vi "ScanFeedback.vi"(2 "measurement type":T1(tab)) -> (1 "V breakdown":dbl, 5 "V depletion":dbl, 6 "Maximum current fluctuations [%]":dbl[](array[numeric]), 8 "Ris [MOhm]":dbl, 9 "Cis @300V [pF/cm]":dbl)   [LabVIEW 2018]
uses:
  globals/QC_MeasurementSetup.vi
  globals/QC_RunInformation.vi
  <vilib>/Analysis/NI_AALPro.lvlib
  <vilib>/Analysis/NI_AALBase.lvlib
panel:
  out "MEAN":dbl
  out "STD":dbl
  out "Index lin fit 1":dbl
  out "Slope":dbl
  out "capSquare1":dbl[](array[numeric])
  out "volts1":dbl[](array[numeric])
  out "volts2":dbl[](array[numeric])
  out "capSquare2":dbl[](array[numeric])
  out "deriv":dbl[](array[numeric])
  out "Slope 2":dbl
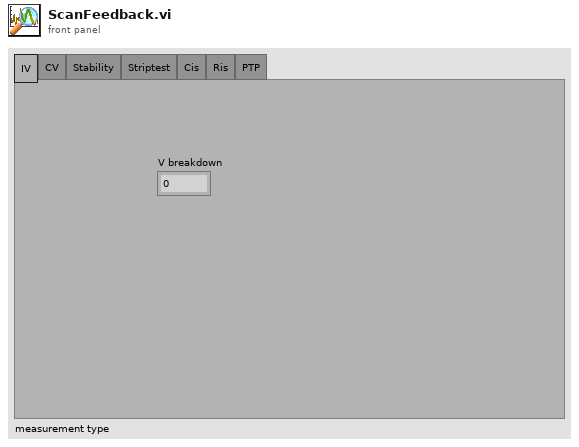
[diagram p1: front panel]
types:
  T1 = enum32{"IV", "CV", "Stability", "Striptest", "Cis", "Ris", "PTP"}
  T2 = enum16{"Reset", "Read Array", "Read Element", "Write Element", "Write Array", "Add Element", "Add Array"}
  T3 = cluster{"Supply":refnum<class "SupplyControl.lvclass">, "Arduino":refnum<class "ArduinoControl.lvclass">, "Measurement switch":refnum<class "Switching.lvclass">, "Initial Voltage [V]":dbl, "Final Voltage [V]":dbl, "Step Size [V]":dbl, "Step Interval [s]":i32, "Number Of Steps":u32, "Ramp down steps [V]":dbl, "Ramp down Interval [s]":i32, "hold steps":i32, "Set Current Limit?":bool, "Current Limit [µA]":dbl, "Temperature Readout":enum16{"Read Arduino", "Enter manually"}, "Supply Name":string, "V_breakdown Limit [V]":dbl, "Measurement switch used?":bool}
  T4 = cluster{"Sensor Serial No.:":string, "Wafer:":string, "Batch:":string, "Manufacturer:":string, "Device Category:":string, "Database Serial No.:":string, "Date Initiated:":string, "Time Initiated:":string, "Test":string, "Probeplan used:":string, "End of Run comment:":string, "User:":string, "Vbias SMU":string, "LCR":string, "Test SMU":string, "Test DMM":string, "Comments":string}
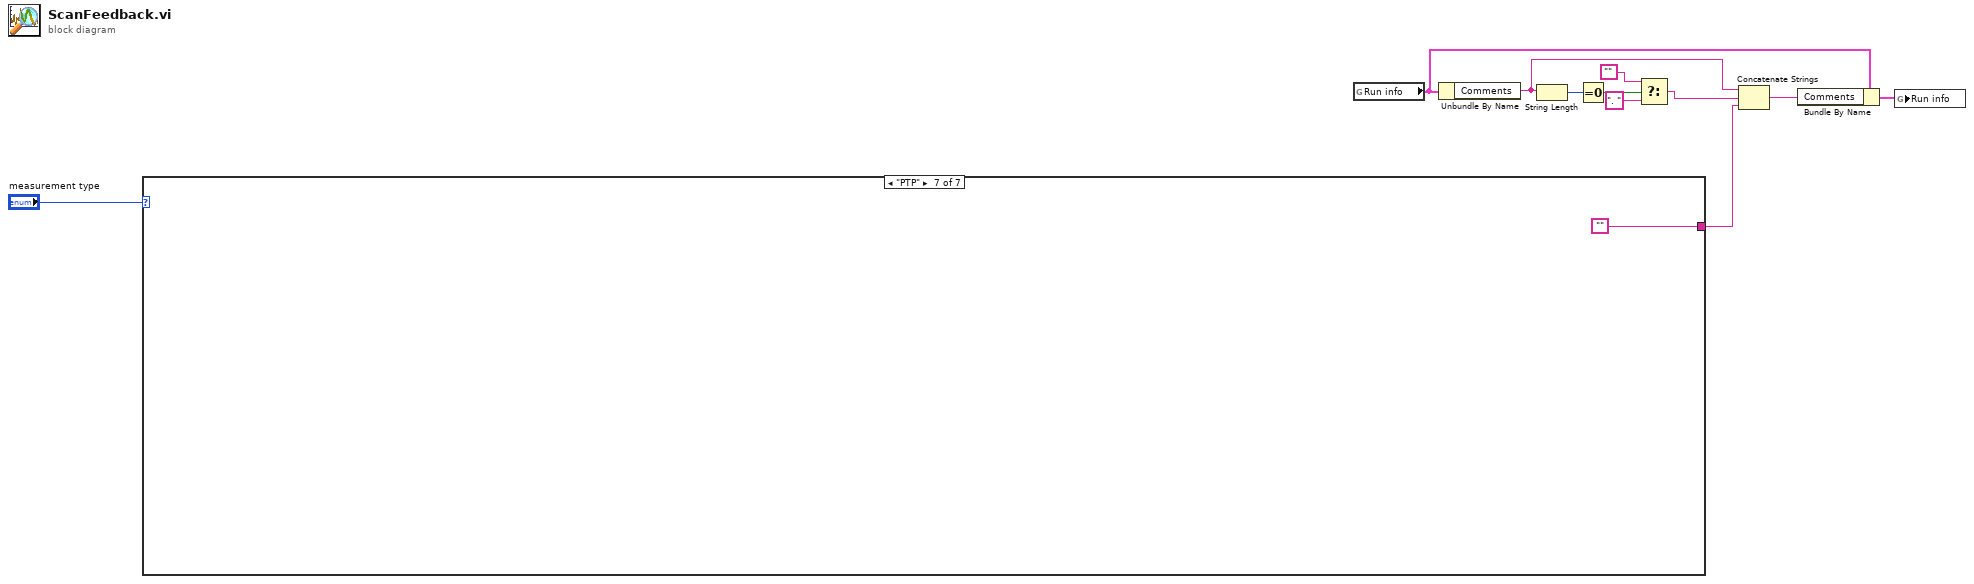
[diagram p0: block diagram]
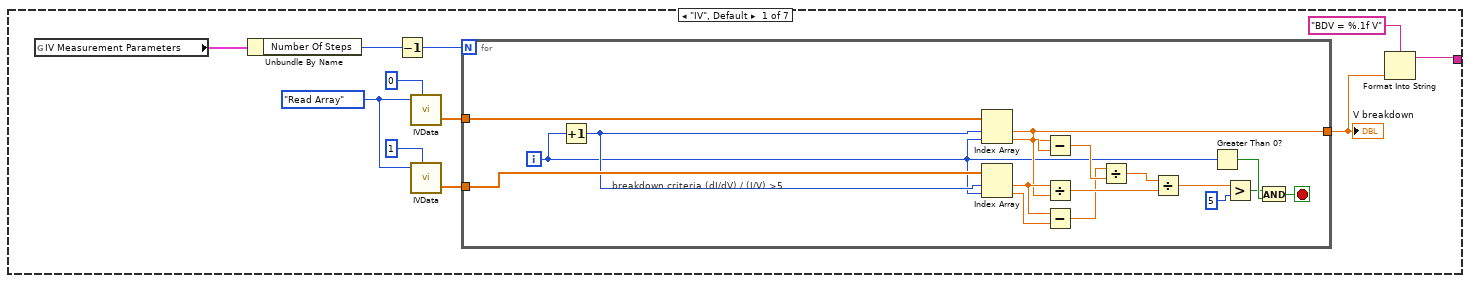
[diagram p2: hidden frame]
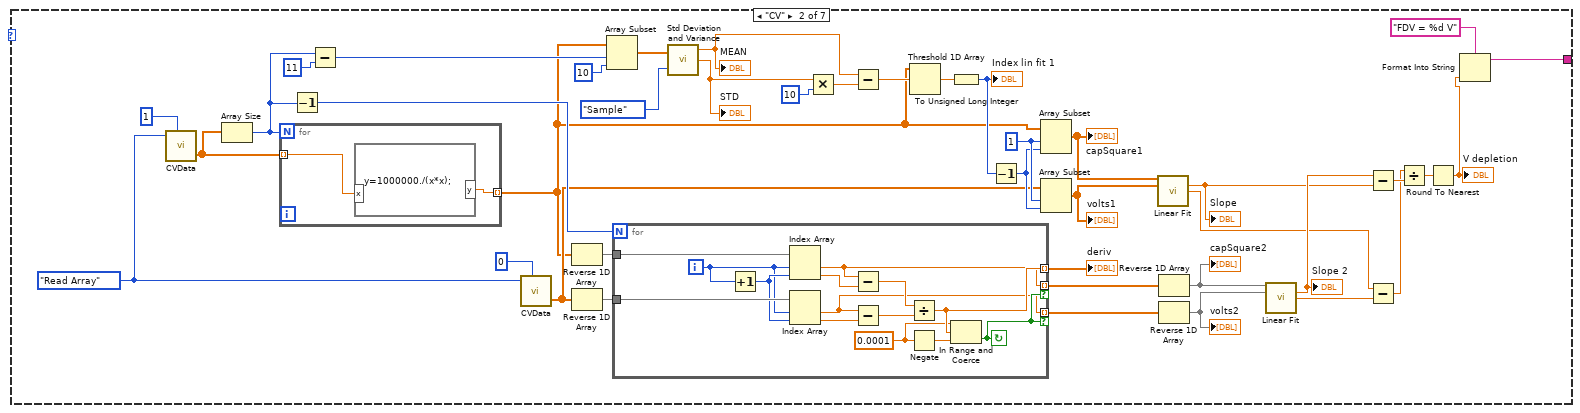
[diagram p3: hidden frame]
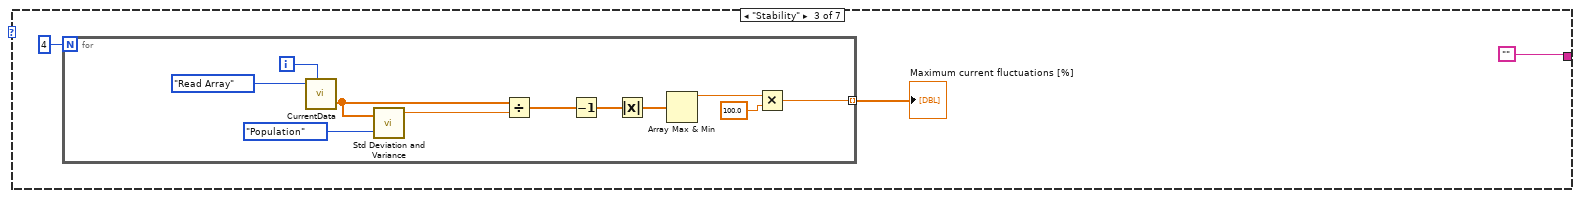
[diagram p4: hidden frame]
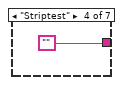
[diagram p5: hidden frame]
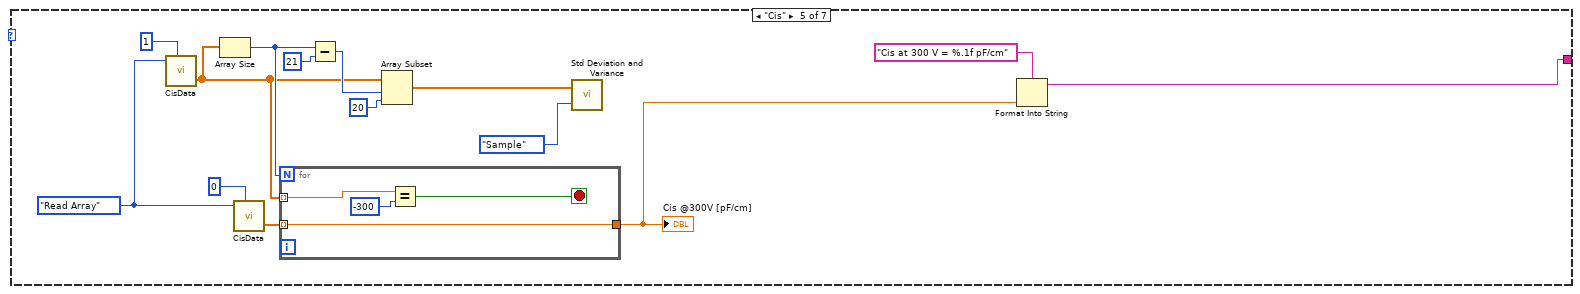
[diagram p6: hidden frame]
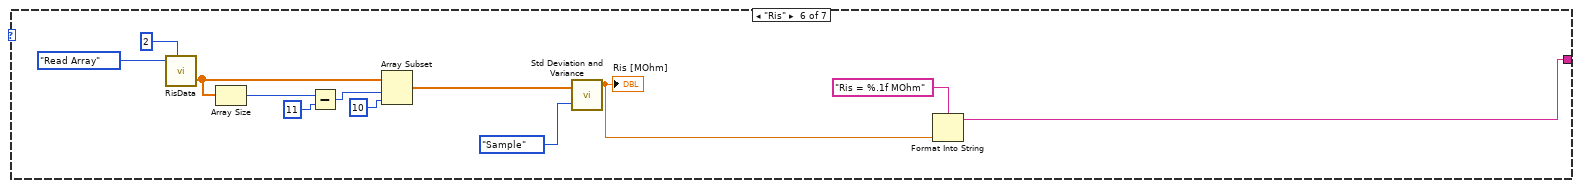
[diagram p7: hidden frame]
diagram:
  n1 = case shown="\"PTP\"" "measurement type" {
    tunnel: [w12 w40 "" "" w112 w130 ""] -> w4
    frame "IV", Default {
      w20 = T2."Read Array" ("Action")
      n2 = global read "QC_MeasurementSetup.vi" "IV Measurement Parameters"() -> (w16:T3)
      n3 = Unbundle By Name(w16) -> ("Number Of Steps"=w15:u32)
      n4 = Decrement(x=w15) -> (x-1=w17:u32)
      n5 = call "IVData.vi"("Action"=w20, "Array No."=0) -> ("Array OUT"=w18:dbl[])  [unwired: 3 in, 1 out]
      n6 = call "IVData.vi"("Action"=w20, "Array No."=1) -> ("Array OUT"=w19:dbl[])  [unwired: 3 in, 1 out]
      n7 = for {
        N: w17 -> [_]
        tunnel: w18 -> [w38]
        tunnel: w19 -> [w39]
        tunnel: [w27] -> w13
        i -> [w25]
        stop <- w23 stop-if-true
        # "breakdown criteria (dI/dV) / (I/V) >5"
        n8 = Increment(x=w25) -> (x+1=w35:i32)
        n9 = Index Array(array=w38, index #1=w35, index #2=w25) -> (element #1=w27:dbl, element #2=w37:dbl)
        n10 = Index Array(array=w39, index #1=w35, index #2=w25) -> (element #1=w30:dbl, element #2=w36:dbl)
        n11 = Subtract(x=w27, y=w37) -> (x-y=w32:dbl)
        n12 = Divide(x=w30, y=w27) -> (x/y=w33:dbl)
        n13 = Subtract(x=w30, y=w36) -> (x-y=w31:dbl)
        n14 = Divide(x=w31, y=w32) -> (x/y=w34:dbl)
        n15 = Divide(x=w34, y=w33) -> (x/y=w28:dbl)
        n16 = Greater Than 0?(x=w25) -> (x > 0?=w26:bool)
        n17 = Greater?(x=w28, y=5) -> (0:w24:bool)
        n18 = And(x=w24, y=w26) -> (x .and. y?=w23:bool)
      }
      "V breakdown" <- w13
      n19 = Format Into String(format string="BDV = %.1f V", w13) -> (resulting string=w12:string)  [unwired: 2 in, 1 out]
    }
    frame "CV" {
      w53 = T2."Read Array" ("Action")
      w50 = 1
      n20 = call "CVData.vi"("Action"=w53, "Array No."=1) -> ("Array OUT"=w44:dbl[])  [unwired: 3 in, 1 out]
      n21 = Array Size(array=w44) -> (size(s)=w45:i32)
      n22 = for {
        N: w45 -> [_]
        tunnel: w44 -> [w82] mode=indexing
        tunnel: [w81] -> w43 mode=indexing
        n23 = formula code="y=1000000./(x*x);"("x"=w82) -> ("y"=w81:dbl)
      }
      n24 = Decrement(x=w45) -> (x-1=w65:i32)
      n25 = Subtract(x=w45, y=11) -> (x-y=w79:i32)
      n26 = call "CVData.vi"("Action"=w53, "Array No."=0) -> ("Array OUT"=w47:dbl[])  [unwired: 3 in, 1 out]
      n27 = Reverse 1D Array(array=w43) -> (reversed array=w68:dbl[])
      n28 = Reverse 1D Array(array=w47) -> (reversed array=w46:dbl[])
      n29 = Array Subset(array=w43, index=w79, length=10) -> (w77:dbl[])
      n30 = for {
        N: w65 -> [_]
        tunnel: w68 -> [w96]
        tunnel: [w89] -> w67 mode=indexing if=w90
        tunnel: [w85] -> w64 mode=indexing if=w90
        tunnel: [w93] -> w61 mode=indexing
        tunnel: w46 -> [w88]
        i -> [w86]
        stop <- w90 continue-if-true
        w91 = 0.0001
        n31 = Increment(x=w86) -> (x+1=w87:i32)
        n32 = Index Array(array=w96, index #1=w86, index #2=w87) -> (element #1=w89:dbl, element #2=w94:dbl)
        n33 = Index Array(array=w88, index #1=w86, index #2=w87) -> (element #1=w85:dbl, element #2=w84:dbl)
        n34 = Subtract(x=w89, y=w94) -> (x-y=w95:dbl)
        n35 = Subtract(x=w85, y=w84) -> (x-y=w83:dbl)
        n36 = Divide(x=w95, y=w83) -> (x/y=w93:dbl)
        n37 = Negate(x=w91) -> (-x=w92:dbl)
        n38 = In Range and Coerce(upper limit=w91, x=w93, lower limit=w92) -> (In Range?=w90:bool)  [unwired: 1 out]
      }
      "deriv" <- w61
      n39 = call <vilib>:"Std Deviation and Variance.vi"("X"=w77, "Weighting (Sample)"=enum16{"Sample", "Population"}."Sample") -> ("mean"=w73:dbl, "standard deviation"=w62:dbl)  [unwired: 1 out]
      "MEAN" <- w73
      "STD" <- w62
      n40 = Multiply(x=w62, y=10) -> (x*y=w74:dbl)
      n41 = Subtract(x=w73, y=w74) -> (x-y=w72:dbl)
      n42 = Threshold 1D Array(2:w72, 3:w43) -> (0:w71:dbl)  [unwired: 1 in]
      n43 = To Unsigned Long Integer(number=w71) -> (unsigned 32bit integer=w70:u32)
      "Index lin fit 1" <- w70
      n44 = Decrement(x=w70) -> (x-1=w49:u32)
      n45 = Array Subset(array=w43, index=w50, length=w49) -> (w69:dbl[])
      "capSquare1" <- w69
      n46 = Array Subset(array=w47, index=w50, length=w49) -> (w48:dbl[])
      "volts1" <- w48
      n47 = call <vilib>:"Linear Fit.vi"("Y"=w69, "X"=w48) -> ("slope"=w59:dbl, "intercept"=w57:dbl)  [unwired: 9 in, 3 out]
      "Slope" <- w59
      n48 = Reverse 1D Array(array=w67) -> (reversed array=w66:dbl[])
      "capSquare2" <- w66
      n49 = Reverse 1D Array(array=w64) -> (reversed array=w63:dbl[])
      "volts2" <- w63
      n50 = call <vilib>:"Linear Fit.vi"("Y"=w66, "X"=w63) -> ("slope"=w60:dbl, "intercept"=w58:dbl)  [unwired: 9 in, 3 out]
      "Slope 2" <- w60
      n51 = Subtract(x=w60, y=w59) -> (x-y=w56:dbl)
      n52 = Subtract(x=w57, y=w58) -> (x-y=w55:dbl)
      n53 = Divide(x=w55, y=w56) -> (x/y=w54:dbl)
      n54 = Round To Nearest(number=w54) -> (nearest integer value=w42:dbl)
      "V depletion" <- w42
      n55 = Format Into String(format string="FDV = %d V", w42) -> (resulting string=w40:string)  [unwired: 2 in, 1 out]
    }
    frame "Stability" {
      n56 = for {
        N: 4 -> [_]
        tunnel: [w100] -> w98 mode=indexing
        i -> [w109]
        n57 = call "CurrentData.vi"("Action"=T2."Read Array", "Array No."=w109) -> ("Array OUT"=w106:dbl[])  [unwired: 3 in, 1 out]
        n58 = call <vilib>:"Std Deviation and Variance.vi"("X"=w106, "Weighting (Sample)"=enum16{"Sample", "Population"}."Population") -> ("mean"=w107:dbl)  [unwired: 2 out]
        n59 = Divide(x=w106, y=w107) -> (x/y=w105:dbl[])
        n60 = Decrement(x=w105) -> (x-1=w104:dbl[])
        n61 = Absolute Value(x=w104) -> (abs(x)=w103:dbl[])
        n62 = Array Max & Min(array=w103) -> (max value=w102:dbl)  [unwired: 3 out]
        n63 = Multiply(x=w102, y=100.0) -> (x*y=w100:dbl)
      }
      "Maximum current fluctuations [%]" <- w98
    }
    frame "Striptest" {
    }
    frame "Cis" {
      w119 = T2."Read Array" ("Action")
      n64 = call "CisData.vi"("Action"=w119, "Array No."=1) -> ("Array OUT"=w116:dbl[])  [unwired: 3 in, 1 out]
      n65 = Array Size(array=w116) -> (size(s)=w117:i32)
      n66 = call "CisData.vi"("Action"=w119, "Array No."=0) -> ("Array OUT"=w115:dbl[])  [unwired: 3 in, 1 out]
      n67 = for {
        N: w117 -> [_]
        tunnel: w116 -> [w128] mode=indexing
        tunnel: w115 -> [w126] mode=indexing
        tunnel: [w126] -> w113
        stop <- w127 stop-if-true
        n68 = Equal?(x=w128, y=-300) -> (x = y?=w127:bool)
      }
      "Cis @300V [pF/cm]" <- w113
      n69 = Subtract(x=w117, y=21) -> (x-y=w121:i32)
      n70 = Array Subset(array=w116, index=w121, length=20) -> (w120:dbl[])
      n71 = call <vilib>:"Std Deviation and Variance.vi"("X"=w120, "Weighting (Sample)"=enum16{"Sample", "Population"}."Sample") -> ()  [unwired: 3 out]
      n72 = Format Into String(format string="Cis at 300 V = %.1f pF/cm", w113) -> (resulting string=w112:string)  [unwired: 2 in, 1 out]
    }
    frame "Ris" {
      n73 = call "RisData.vi"("Action"=T2."Read Array", "Array No."=2) -> ("Array OUT"=w133:dbl[])  [unwired: 3 in, 1 out]
      n74 = Array Size(array=w133) -> (size(s)=w140:i32)
      n75 = Subtract(x=w140, y=11) -> (x-y=w137:i32)
      n76 = Array Subset(array=w133, index=w137, length=10) -> (w136:dbl[])
      n77 = call <vilib>:"Std Deviation and Variance.vi"("X"=w136, "Weighting (Sample)"=enum16{"Sample", "Population"}."Sample") -> ("mean"=w131:dbl)  [unwired: 2 out]
      "Ris [MOhm]" <- w131
      n78 = Format Into String(format string="Ris = %.1f MOhm", w131) -> (resulting string=w130:string)  [unwired: 2 in, 1 out]
    }
    frame "PTP" {
    }
  }
  n79 = global read "QC_RunInformation.vi" "Run info"() -> (w3:T4)
  n80 = Unbundle By Name(w3) -> ("Comments"=w6:string)
  n81 = String Length(string=w6) -> (length=w10:i32)
  n82 = Equal To 0?(x=w10) -> (x = 0?=w9:bool)
  n83 = Select(t="", s=w9, f=". ") -> (s? t:f=w5:string)
  n84 = Concatenate Strings(w6, w5, w4) -> (w2:string)
  n85 = Bundle By Name(cluster=w3, "Comments"=w2) -> (w1:T4)
  n86 = global write "QC_RunInformation.vi" "Run info"(w1) -> ()
